vi "Start cycling.vi"(8 "error in":errorcluster, 9 "Cycling interval":dbl=500.0 format="%#_gms", 10 "Triggered interval":dbl=500.0 format="%#_gms") -> (0 "error out":errorcluster)   [LabVIEW 2020, in "Cycling by State module.lvlib"]
doc: "To start cycling by waking up cycling helper loop\n_____\nCreated using DQMH Event Scripter 7.0.1.1316."
uses:
  Cycling by State module.lvlib
  Start cycling Argument--cluster.ctl
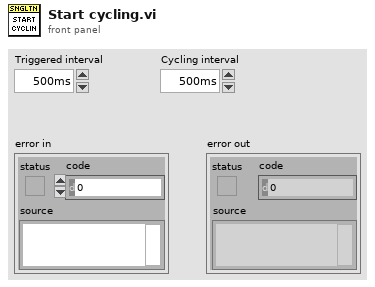
[diagram p1: front panel]
types:
  T1 = typedef "Cycling by State module.lvlib/Start cycling Argument--cluster.ctl" = cluster{"Triggered interval":dbl, "Cycling interval":dbl}
  T2 = typedef "Cycling by State module.lvlib/Request Events--cluster.ctl" = cluster{"Stop Module":refnum<user-event>, "Show Panel":refnum<user-event>, "Hide Panel":refnum<user-event>, "Get Module Execution Status":refnum<user-event>, "Show Diagram":refnum<user-event>, "Start cycling":refnum<user-event>, "Stop cycling":refnum<user-event>, "Private":cluster{"Wake up cycling HL":refnum<user-event>}}
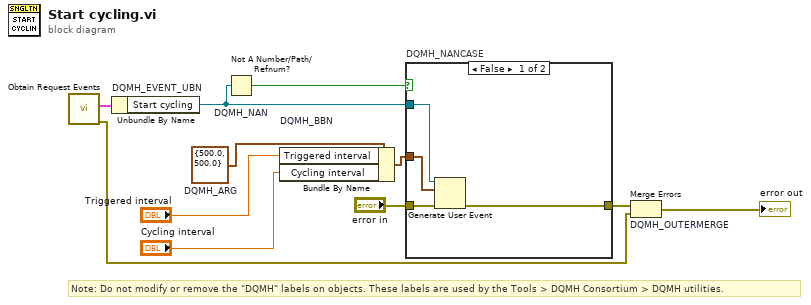
[diagram p0: block diagram]
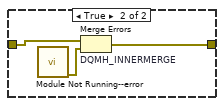
[diagram p2: hidden frame]
diagram:
  w5 = T1 {"Triggered interval"=500.0, "Cycling interval"=500.0}  # DQMH_ARG
  # "Note: Do not modify or remove the \"DQMH\" labels on objects. These labels are used by the Tools > DQMH Consortium > DQMH utilities."
  n1 = call "Obtain Request Events.vi"() -> ("error out"=w3:errorcluster, "Cycling by State module Request Events"=w2:T2)  [unwired: 10 in]
  n2 = Unbundle By Name "DQMH_EVENT_UBN"(w2) -> ("Start cycling"=w7:refnum<user-event>)
  n3 = Not A Number/Path/Refnum? "DQMH_NAN"(number/path/refnum=w7) -> (NaN/Path/Refnum?=w8:bool)
  n4 = Bundle By Name "DQMH_BBN"(cluster=w5, "Triggered interval"="Triggered interval", "Cycling interval"="Cycling interval") -> (w9:T1)
  n5 = case "DQMH_NANCASE" shown="False" w8 {
    tunnel: "error in" -> [w15 w18]
    tunnel: [w14 w17] -> w6
    tunnel: w7 -> [w13 _]
    tunnel: w9 -> [w12 _]
    frame False {
      n6 = Generate User Event(user event=w13, event data cluster=w12, error in=w15) -> (error out=w14:errorcluster)  [unwired: 1 in, 1 out]
    }
    frame True {
      n7 = call "Module Not Running--error.vi"() -> ("error out"=w16:errorcluster)  [unwired: 11 in]
      n8 = Merge Errors "DQMH_INNERMERGE"(w18, w16) -> (w17:errorcluster)
    }
  }
  n9 = Merge Errors "DQMH_OUTERMERGE"(w6, w3) -> (→"error out":errorcluster)
